vi "decimate magnetomer array.vi"(10 "new size":i32=25, 11 "orbit magnetic field data":T1 {"omega" format="%#_13g"}) -> (3 "orbit magnetic field data 2":T1 {"omega" format="%#_13g"})   [LabVIEW 2017]
uses:
  typedefs/orbit magnetic field data.ctl
  typedefs/magnetomter reading set.ctl
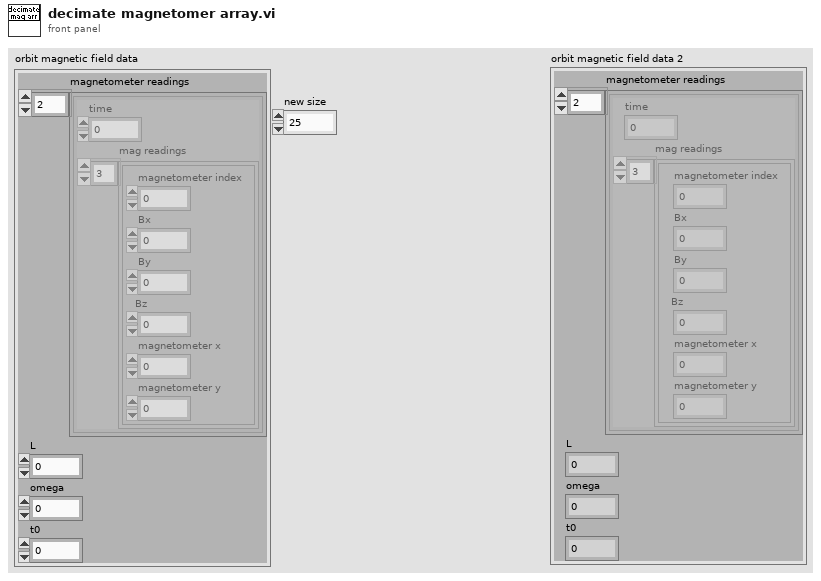
[diagram p1: front panel]
types:
  T1 = typedef "orbit magnetic field data.ctl" = cluster{"magnetometer readings":T2[], "L":dbl, "omega":dbl, "t0":dbl}
  T2 = typedef "magnetomter reading set.ctl" = cluster{"time":fxp<+,48,48>, "mag readings":cluster{"magnetometer index":dbl, "Bx":dbl, "By":dbl, "Bz":dbl, "magnetometer x":dbl, "magnetometer y":dbl}[]}
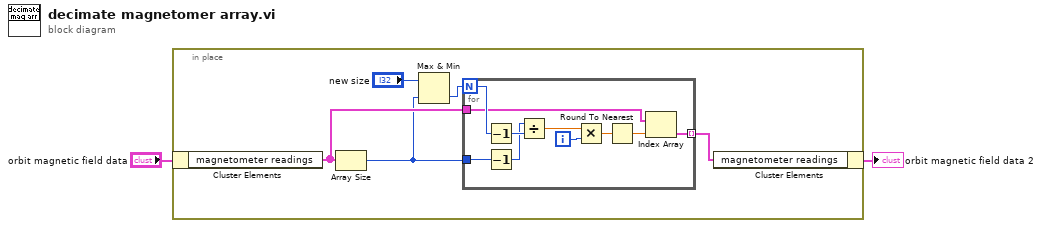
[diagram p0: block diagram]
diagram:
  n1 = in-place {
    n2 = in-place-cluster #1("orbit magnetic field data") -> ("magnetometer readings"=w7:T2[])
    n3 = Array Size(array=w7) -> (size(s)=w3:i32)
    n4 = Max & Min(x="new size", y=w3) -> (min(x,y)=w4:i32)  [unwired: 1 out]
    n5 = for {
      N: w4 -> [w17]
      tunnel: w7 -> [w12]
      tunnel: [w9] -> w6 mode=indexing
      tunnel: w3 -> [w8]
      i -> [w15]
      n6 = Decrement(x=w17) -> (x-1=w14:i32)
      n7 = Decrement(x=w8) -> (x-1=w13:i32)
      n8 = Divide(x=w13, y=w14) -> (x/y=w16:dbl)
      n9 = Multiply(x=w16, y=w15) -> (x*y=w11:dbl)
      n10 = Round To Nearest(number=w11) -> (nearest integer value=w10:dbl)
      n11 = Index Array(array=w12, index=w10) -> (element=w9:T2)
    }
    n12 = in-place-cluster #1("magnetometer readings"=w6) -> (→"orbit magnetic field data 2":T1)
  }
